vi "StopAllWaveforms.vi"(11 "Handle":u64) -> (3 "FT_Status":u64(ring) items=["FT_OK", "FT_INVALID_HANDLE", "FT_DEVICE_NOT_FOUND", "FT_DEVICE_NOT_OPENED", "FT_IO_ERROR", "FT_INSUFFICIENT_RESOURCES", "FT_INVALID_PARAMETER", "FT_INVALID_BAUD_RATE", "FT_DEVICE_NOT_OPENED_FOR_ERASE", "FT_DEVICE_NOT_OPENED_FOR_WRITE", "FT_FAILED_TO_WRITE_DEVICE", "FT_EEPROM_READ_FAILED", "FT_EEPROM_WRITE_FAILED", "FT_EEPROM_ERASE_FAILED", "FT_EEPROM_NOT_PRESENT", "FT_EEPROM_NOT_PROGRAMMED", "FT_INVALID_ARGS", "FT_NOT_SUPPORTED", "FT_OTHER_ERROR"])   [LabVIEW 2017]
panel:
  out "Bytes Written":u64
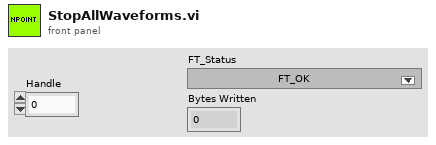
[diagram p1: front panel]
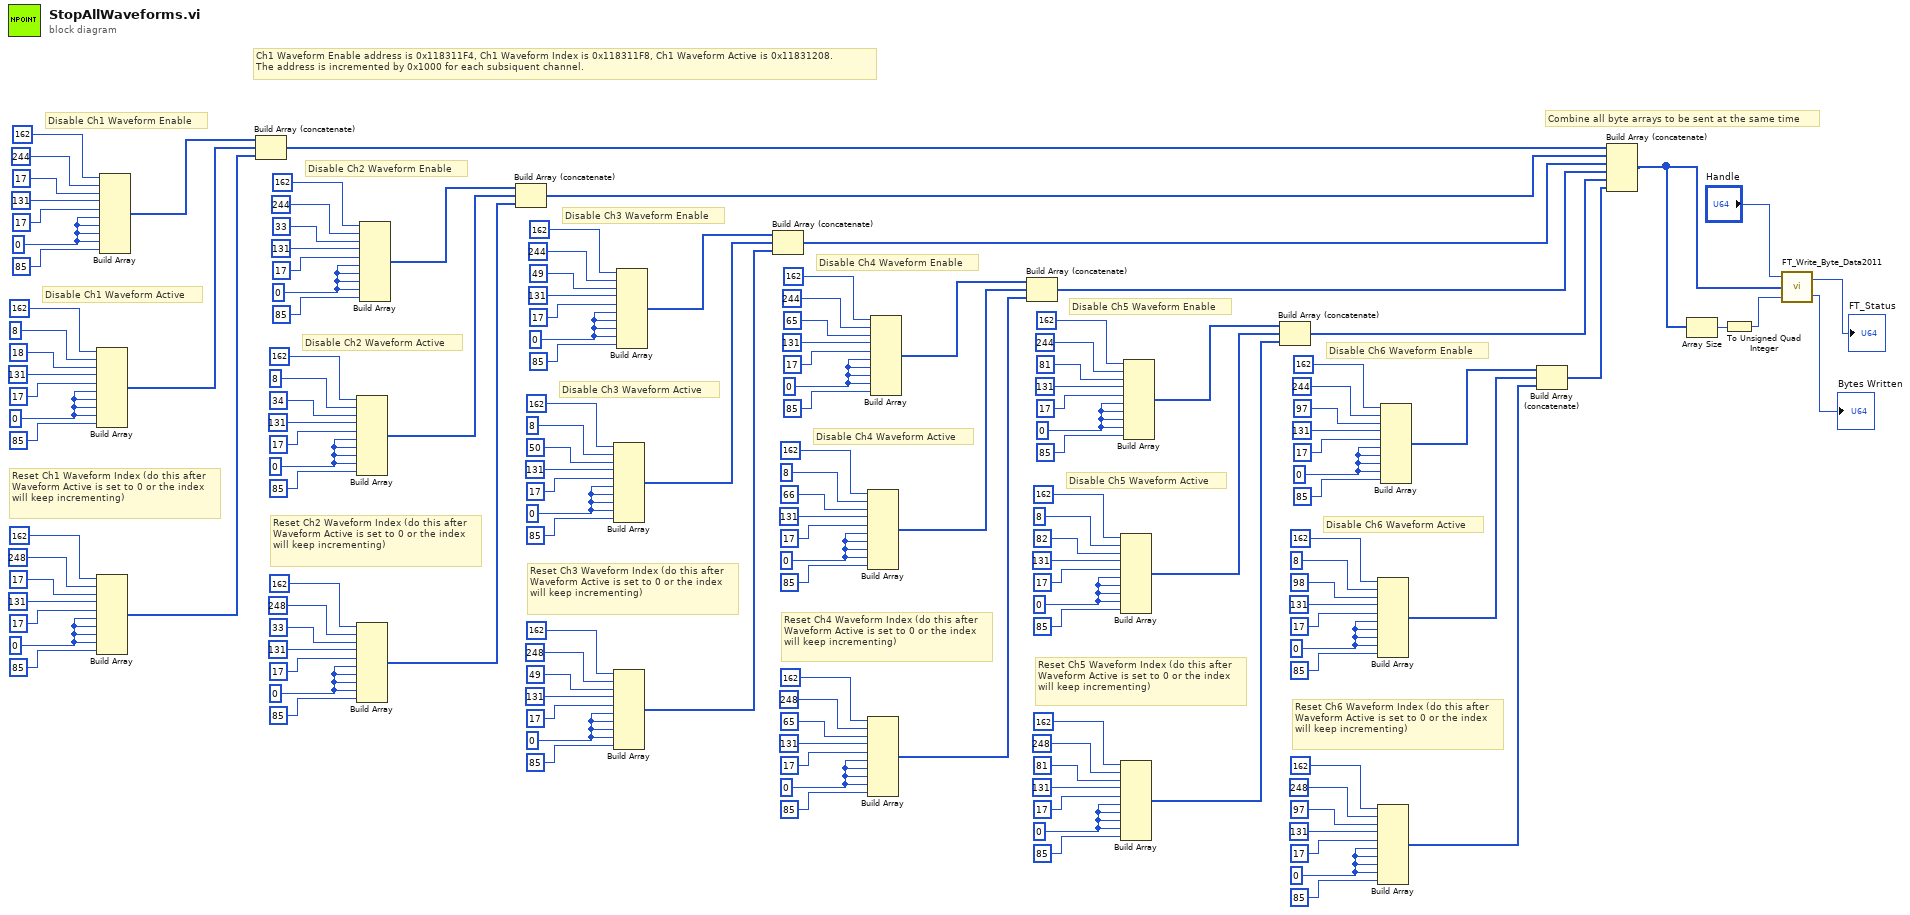
[diagram p0: block diagram]
diagram:
  w9 = u8 0 ("element")
  w17 = u8 0 ("element")
  w24 = u8 0 ("element")
  w33 = u8 0 ("element")
  w41 = u8 0 ("element")
  w48 = u8 0 ("element")
  w57 = u8 0 ("element")
  w65 = u8 0 ("element")
  w72 = u8 0 ("element")
  w81 = u8 0 ("element")
  w89 = u8 0 ("element")
  w96 = u8 0 ("element")
  w105 = u8 0 ("element")
  w113 = u8 0 ("element")
  w120 = u8 0 ("element")
  w129 = u8 0 ("element")
  w137 = u8 0 ("element")
  w144 = u8 0 ("element")
  # "Combine all byte arrays to be sent at the same time"
  # "Reset Ch6 Waveform Index (do this after Waveform Active is set to 0 or the index will keep incrementing)"
  # "Disable Ch6 Waveform Active"
  # "Disable Ch6 Waveform Enable"
  # "Reset Ch5 Waveform Index (do this after Waveform Active is set to 0 or the index will keep incrementing)"
  # "Disable Ch5 Waveform Active"
  # "Disable Ch5 Waveform Enable"
  # "Reset Ch4 Waveform Index (do this after Waveform Active is set to 0 or the index will keep incrementing)"
  # "Disable Ch4 Waveform Active"
  # "Disable Ch4 Waveform Enable"
  # "Reset Ch3 Waveform Index (do this after Waveform Active is set to 0 or the index will keep incrementing)"
  # "Disable Ch3 Waveform Active"
  # "Disable Ch3 Waveform Enable"
  # "Reset Ch2 Waveform Index (do this after Waveform Active is set to 0 or the index will keep incrementing)"
  # "Disable Ch2 Waveform Active"
  # "Disable Ch2 Waveform Enable"
  # "Reset Ch1 Waveform Index (do this after Waveform Active is set to 0 or the index will keep incrementing)"
  # "Disable Ch1 Waveform Active"
  # "Disable Ch1 Waveform Enable"
  # "Ch1 Waveform Enable address is 0x118311F4, Ch1 Waveform Index is 0x118311F8, Ch1 Waveform Active is 0x11831208.\nThe address is incremented by 0x1000 for each subsiquent channel."
  n1 = Build Array(u8 162 ("element"), u8 8 ("element"), u8 18 ("element"), u8 131 ("element"), u8 17 ("element"), w137, w137, w137, w137, u8 85 ("element")) -> (w136:u8[])
  n2 = Build Array(u8 162 ("element"), u8 248 ("element"), u8 17 ("element"), u8 131 ("element"), u8 17 ("element"), w129, w129, w129, w129, u8 85 ("element")) -> (w128:u8[])
  n3 = Build Array(u8 162 ("element"), u8 244 ("element"), u8 17 ("element"), u8 131 ("element"), u8 17 ("element"), w144, w144, w144, w144, u8 85 ("element")) -> (w150:u8[])
  n4 = Build Array (concatenate)(w150, w136, w128) -> (w7:u8[])
  n5 = Build Array(u8 162 ("element"), u8 8 ("element"), u8 34 ("element"), u8 131 ("element"), u8 17 ("element"), w113, w113, w113, w113, u8 85 ("element")) -> (w112:u8[])
  n6 = Build Array(u8 162 ("element"), u8 248 ("element"), u8 33 ("element"), u8 131 ("element"), u8 17 ("element"), w105, w105, w105, w105, u8 85 ("element")) -> (w104:u8[])
  n7 = Build Array(u8 162 ("element"), u8 244 ("element"), u8 33 ("element"), u8 131 ("element"), u8 17 ("element"), w120, w120, w120, w120, u8 85 ("element")) -> (w123:u8[])
  n8 = Build Array (concatenate)(w123, w112, w104) -> (w6:u8[])
  n9 = Build Array(u8 162 ("element"), u8 8 ("element"), u8 50 ("element"), u8 131 ("element"), u8 17 ("element"), w89, w89, w89, w89, u8 85 ("element")) -> (w88:u8[])
  n10 = Build Array(u8 162 ("element"), u8 248 ("element"), u8 49 ("element"), u8 131 ("element"), u8 17 ("element"), w81, w81, w81, w81, u8 85 ("element")) -> (w80:u8[])
  n11 = Build Array(u8 162 ("element"), u8 244 ("element"), u8 49 ("element"), u8 131 ("element"), u8 17 ("element"), w96, w96, w96, w96, u8 85 ("element")) -> (w99:u8[])
  n12 = Build Array (concatenate)(w99, w88, w80) -> (w5:u8[])
  n13 = Build Array(u8 162 ("element"), u8 8 ("element"), u8 66 ("element"), u8 131 ("element"), u8 17 ("element"), w65, w65, w65, w65, u8 85 ("element")) -> (w64:u8[])
  n14 = Build Array(u8 162 ("element"), u8 248 ("element"), u8 65 ("element"), u8 131 ("element"), u8 17 ("element"), w57, w57, w57, w57, u8 85 ("element")) -> (w56:u8[])
  n15 = Build Array(u8 162 ("element"), u8 244 ("element"), u8 65 ("element"), u8 131 ("element"), u8 17 ("element"), w72, w72, w72, w72, u8 85 ("element")) -> (w75:u8[])
  n16 = Build Array (concatenate)(w75, w64, w56) -> (w4:u8[])
  n17 = Build Array(u8 162 ("element"), u8 8 ("element"), u8 82 ("element"), u8 131 ("element"), u8 17 ("element"), w41, w41, w41, w41, u8 85 ("element")) -> (w40:u8[])
  n18 = Build Array(u8 162 ("element"), u8 248 ("element"), u8 81 ("element"), u8 131 ("element"), u8 17 ("element"), w33, w33, w33, w33, u8 85 ("element")) -> (w32:u8[])
  n19 = Build Array(u8 162 ("element"), u8 244 ("element"), u8 81 ("element"), u8 131 ("element"), u8 17 ("element"), w48, w48, w48, w48, u8 85 ("element")) -> (w51:u8[])
  n20 = Build Array (concatenate)(w51, w40, w32) -> (w3:u8[])
  n21 = Build Array(u8 162 ("element"), u8 8 ("element"), u8 98 ("element"), u8 131 ("element"), u8 17 ("element"), w17, w17, w17, w17, u8 85 ("element")) -> (w16:u8[])
  n22 = Build Array(u8 162 ("element"), u8 248 ("element"), u8 97 ("element"), u8 131 ("element"), u8 17 ("element"), w9, w9, w9, w9, u8 85 ("element")) -> (w8:u8[])
  n23 = Build Array(u8 162 ("element"), u8 244 ("element"), u8 97 ("element"), u8 131 ("element"), u8 17 ("element"), w24, w24, w24, w24, u8 85 ("element")) -> (w27:u8[])
  n24 = Build Array (concatenate)(w27, w16, w8) -> (w2:u8[])
  n25 = Build Array (concatenate)(w7, w6, w5, w4, w3, w2) -> (w1:u8[])
  n26 = Array Size(array=w1) -> (size(s)=w156:i32)
  n27 = To Unsigned Quad Integer(1:w156) -> (0:w155:u64)
  n28 = call "FT_Write_Byte_Data2011.vi"("Bytes To Write"=w155, "Buffer"=w1, "Handle"="Handle") -> ("Bytes Written"=→"Bytes Written":u64, "FT_Status"=→"FT_Status":u64)
